vi "Tosca-Setup Connections.vi"(0 "Connect":T2, 2 "Parent VI":refnum<vi>, 7 "config path":path) -> (4 "Connect out":T2, 8 "Canceled?":bool)   [LabVIEW 2020]
uses:
  Classes/Parameters/Connect.ctl
  epl-vi-lib/Utility VIs/Buttons/KCheckmarkBoolean 2.ctl
  Typedefs/Tosca-Locomotion Settings.ctl
  epl-vi-lib/PXI DAQ VIs/TDT VIs/TDT ET VIs/TDT ET-Command Enum.ctl
  epl-vi-lib/TCP VIs/TCP Params.ctl
  epl-vi-lib/TCP VIs/TCP Write.vi
  epl-vi-lib/TCP VIs/TCP-Check Result.vi
  Classes/Parameters/Parameters.lvclass
panel:
  in  "Codes":string
  in  "TCP markers":bool
  in  "LocoTCP":string
  in  "Retrieve data":T1
  in  "Loco Test":cluster{"Ping":bool, "Result":bool}
  in  "Pupil Test":cluster{"Ping":bool, "Result":bool}
  in  "Loco":T1 caption="Record locomotion data"
  in  "Pupil?":T1 caption="Record video"
  out "Ping result":bool
  in  "Ping":bool
  in  "SMP?":T1 caption="Record significant motion pixels (SMP)"
  in  "ET?":T1 caption="Interface with Synapse"
  in  "Cancel":bool
  in  "Apply":bool
  # "Webcam"
  # "Vision display"
  # "Video"
  # "Locomotion"
  # "Neural data"
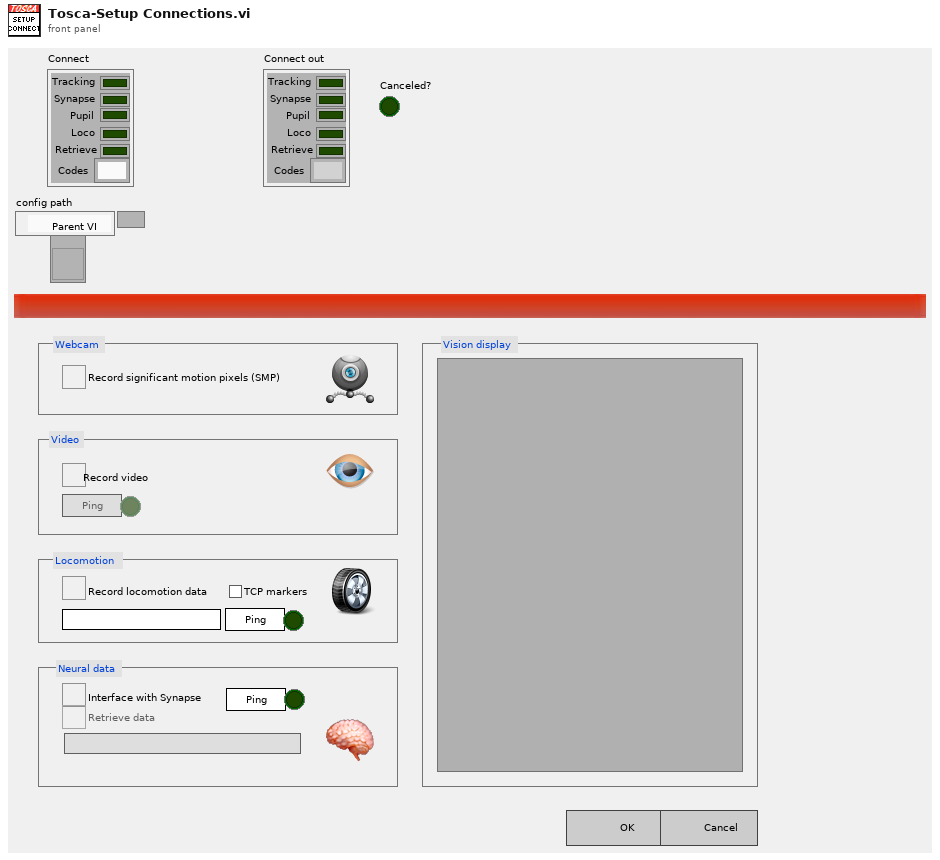
[diagram p1: front panel]
types:
  T1 = typedef "KCheckmarkBoolean 2.ctl" = bool
  T2 = typedef "Parameters.lvclass/Connect.ctl" = cluster{"Tracking":bool, "Synapse":bool, "Pupil":bool, "Loco":bool, "Retrieve":bool, "Codes":string}
  T3 = typedef "TDT ET-Command Enum.ctl" = enum16{"Ping", "Start", "Stop", "NewBlock"}
  T4 = typedef "Tosca-Locomotion Settings.ctl" = cluster{"IP Address":string, "Port":i32, "Send markers":bool}
  T5 = enum8{"Enabled", "Disabled", "Disabled and Grayed Out"}
  T6 = typedef "TCP Params.ctl" = cluster{"IP Address":string, "Port":i32}
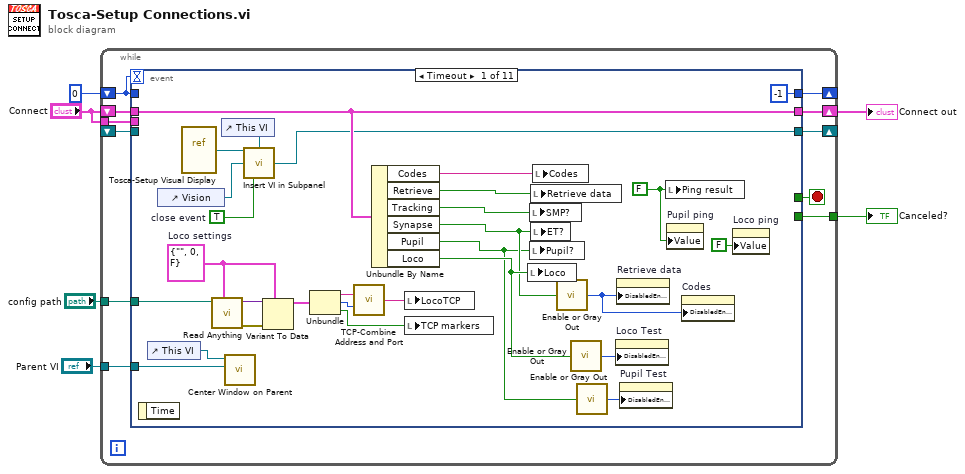
[diagram p0: block diagram]
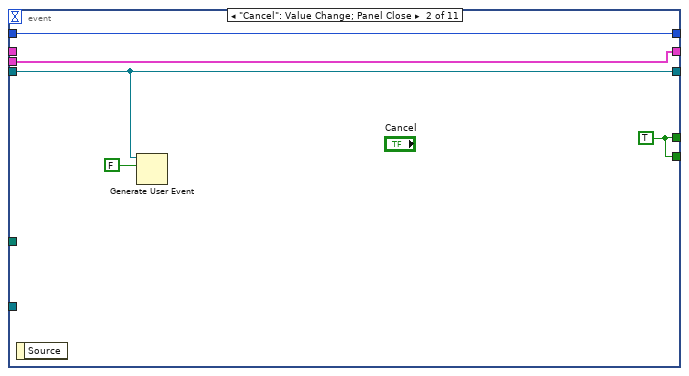
[diagram p2: hidden frame]
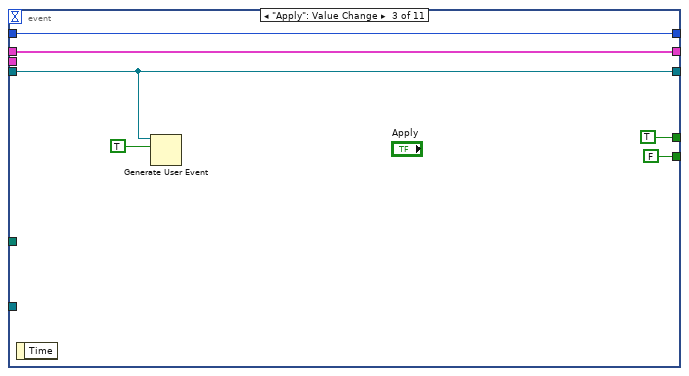
[diagram p3: hidden frame]
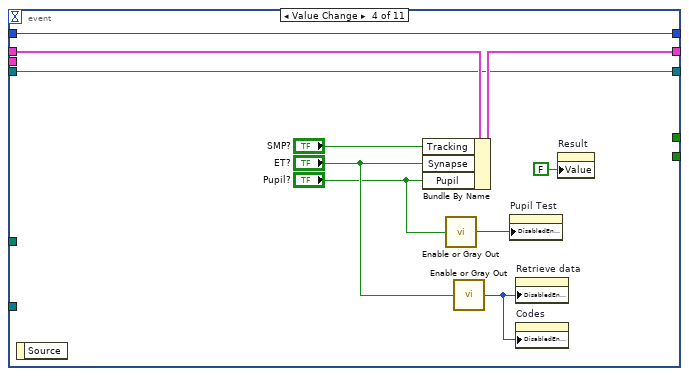
[diagram p4: hidden frame]
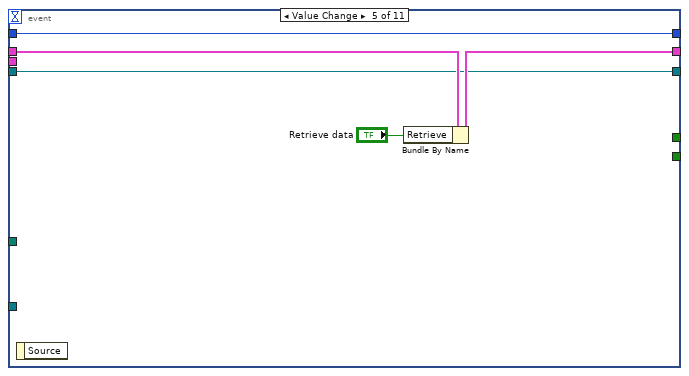
[diagram p5: hidden frame]
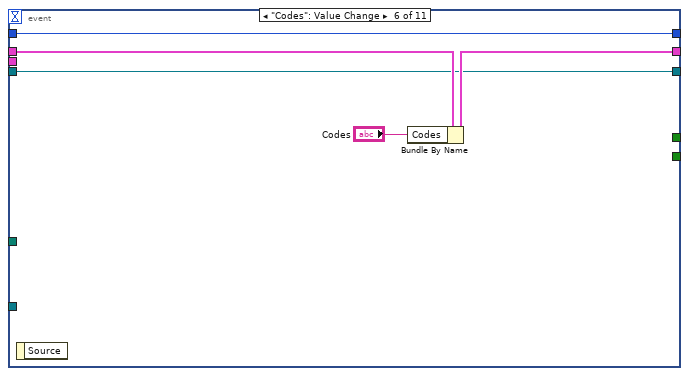
[diagram p6: hidden frame]
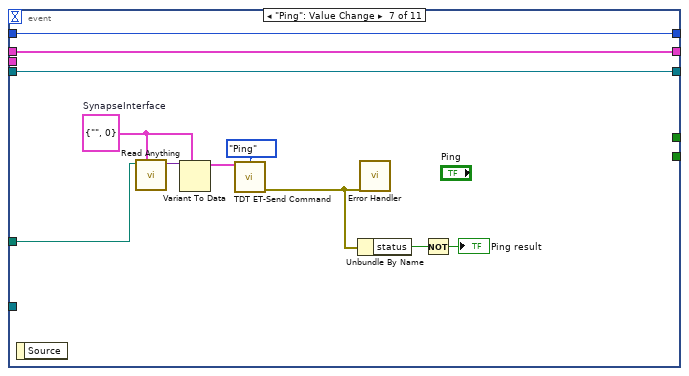
[diagram p7: hidden frame]
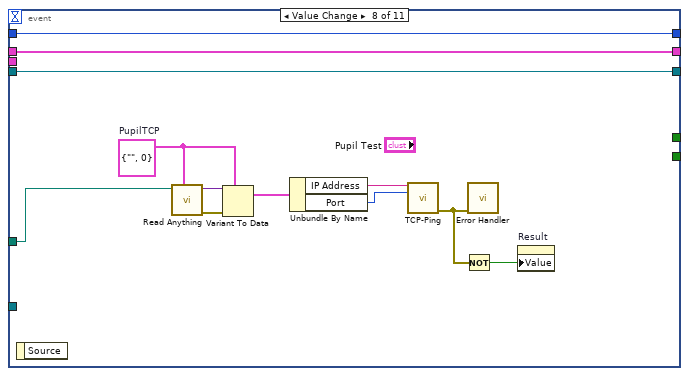
[diagram p8: hidden frame]
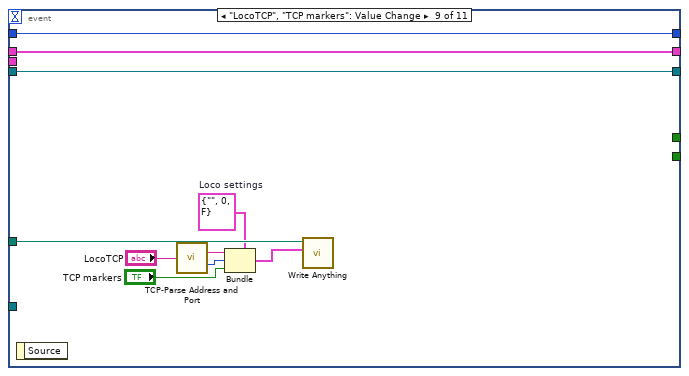
[diagram p9: hidden frame]
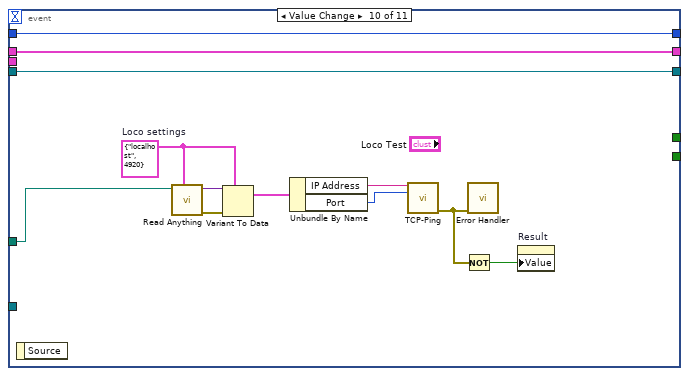
[diagram p10: hidden frame]
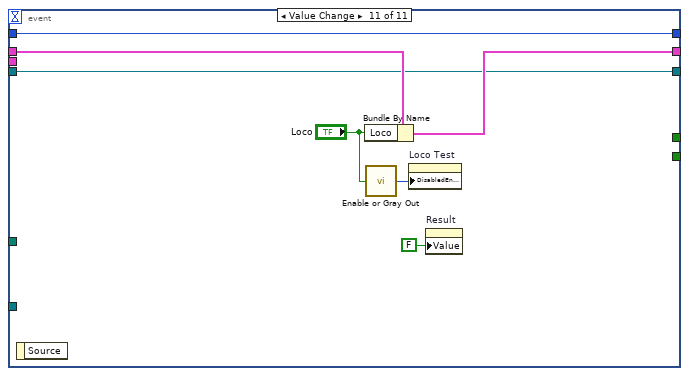
[diagram p11: hidden frame]
diagram:
  n1 = while {
    shift-right: [w17] -> _
    shift-left: 0 -> [w10]
    tunnel: [w13] -> w4
    shift-right: [w15] -> w5
    shift-left: "Connect" -> [w16]
    tunnel: "config path" -> [w12]
    tunnel: "Connect" -> [w11]
    tunnel: "Parent VI" -> [w9]
    shift-right: [w8] -> _
    shift-left: _ -> [w7]
    stop <- w14 stop-if-true
    n2 = event shown="[0] Timeout" {
      selector: _ -> [_ _ _ _ _ _ _ _ _ _ _]
      dyn-events: _ -> [_ _ _ _ _ _ _ _ _ _ _]
      timeout: w10 -> [_ _ _ _ _ _ _ _ _ _ _]
      tunnel: [-1 w49 w54 w64 w72 w77 w83 w100 w110 w122 w129] -> w17
      tunnel: w16 -> [w45 _ w57 w67 w71 w76 w88 w99 w109 w121 w128]
      tunnel: [w45 w50 w57 w66 w70 w75 w88 w99 w109 w121 w127] -> w15
      tunnel: [_ w51 TRUE _ _ _ _ _ _ _ _] -> w14
      tunnel: [_ w51 FALSE _ _ _ _ _ _ _ _] -> w13
      tunnel: w12 -> [w22 _ _ _ _ _ w79 w90 w104 w112 _]
      tunnel: w11 -> [_ w50 _ _ _ _ _ _ _ _ _]
      tunnel: w10 -> [_ w49 w54 w64 w72 w77 w83 w100 w110 w122 w129]
      tunnel: w9 -> [w35 _ _ _ _ _ _ _ _ _ _]
      tunnel: [w29 w48 w53 w59 w68 w74 w82 w89 w108 w111 w123] -> w8
      tunnel: w7 -> [_ w48 w53 w59 w68 w74 w82 w89 w108 w111 w123]
      event Timeout {
        w21 = T4 {"IP Address"="", "Port"=0, "Send markers"=FALSE}  # Loco settings
        w30 = TRUE  # close event
        w40 = FALSE ("Ping result")
        n3 = event-data() -> ()  [unwired: 1 in, 1 out]
        n4 = control-ref of="This VI"() -> (w34:refnum<vi>)
        n5 = control-ref of="Vision"() -> (w32:refnum<vi>)
        n6 = vi-ref "Tosca-Setup Visual Display.vi"() -> (w33:refnum<vi>)
        n7 = call "Read Anything.vi"("Type of Anything"=w21, "Path (dialog)"=w22) -> ("Error Out"=w28:errorcluster, "Anything"=w27:variant)  [unwired: 7 in, 1 out]
        n8 = control-ref of="This VI"() -> (w31:refnum<vi>)
        n9 = call "Center Window on Parent.vi"("Parent VI"=w35, "VI in"=w34) -> ()  [unwired: 8 in, 2 out]
        n10 = call "Insert VI in Subpanel.vi"("VI Ref"=w33, "Parent"=w31, "SubPanel"=w32, "close event"=w30) -> ("close event"=w29:refnum<user-event>)  [unwired: 10 in, 1 out]
        n11 = Variant To Data(error in=w28, type=w21, Variant=w27) -> (data=w26:T4)  [unwired: 1 out]
        n12 = Unbundle(w26) -> ("IP Address"=w25:string, "Port"=w23:i32, "Send markers"=w20:bool)
        n13 = call "TCP-Combine Address and Port.vi"("Address"=w25, "Port"=w23) -> ("Address out"=w24:string)  [unwired: 13 in]
        n14 = Unbundle By Name(w45) -> ("Codes"=w18:string, "Retrieve"=w37:bool, "Tracking"=w44:bool, "Synapse"=w38:bool, "Pupil"=w36:bool, "Loco"=w42:bool)
        n15 = local write "LocoTCP"(w24) -> ()
        n16 = local write "TCP markers"(w20) -> ()
        n17 = local write "Loco"(w42) -> ()
        n18 = local write "SMP?"(w44) -> ()
        n19 = local write "Pupil?"(w36) -> ()
        n20 = local write "Retrieve data"(w37) -> ()
        n21 = local write "ET?"(w38) -> ()
        n22 = local write "Codes"(w18) -> ()
        n23 = call "Enable or Gray Out.vi"("Boolean"=w38) -> ("Disabled"=w19:T5)
        n24 = call "Enable or Gray Out.vi"("Boolean"=w42) -> ("Disabled"=w43:T5)
        n25 = call "Enable or Gray Out.vi"("Boolean"=w36) -> ("Disabled"=w41:T5)
        n26 = property on="Loco Test" class="Clust"("DisabledEnum"=w43) -> ()  [unwired: 2 in, 2 out]
        n27 = property on="Retrieve data" class="Bool (strict)"("DisabledEnum"=w19) -> ()  [unwired: 2 in, 2 out]
        n28 = property on="Pupil Test" class="Clust"("DisabledEnum"=w41) -> ()  [unwired: 2 in, 2 out]
        n29 = local write "Ping result"(w40) -> ()
        n30 = property on="Pupil ping" class="Bool (strict)"("Value"=w40) -> ()  [unwired: 2 in, 2 out]
        n31 = property on="Codes" class="Str"("DisabledEnum"=w19) -> ()  [unwired: 2 in, 2 out]
        n32 = property on="Loco ping" class="Bool (strict)"("Value"=FALSE) -> ()  [unwired: 2 in, 2 out]
      }
      event "Cancel": Value Change; Panel Close {
        w51 = TRUE
        n33 = event-data() -> ()  [unwired: 1 in, 1 out]
        n34 = Generate User Event(user event=w48, event data cluster=FALSE ("event data")) -> ()  [unwired: 2 in, 2 out]
      }
      event "Apply": Value Change {
        n35 = event-data() -> ()  [unwired: 1 in, 1 out]
        n36 = Generate User Event(user event=w53, event data cluster=TRUE ("event data")) -> ()  [unwired: 2 in, 2 out]
      }
      event Value Change {
        n37 = event-data() -> ()  [unwired: 1 in, 1 out]
        n38 = Bundle By Name(cluster=w67, "Tracking"="SMP?", "Synapse"="ET?", "Pupil"="Pupil?") -> (w66:T2)
        n39 = call "Enable or Gray Out.vi"("Boolean"="Pupil?") -> ("Disabled"=w63:T5)
        n40 = call "Enable or Gray Out.vi"("Boolean"="ET?") -> ("Disabled"=w58:T5)
        n41 = property on="Pupil Test" class="Clust"("DisabledEnum"=w63) -> ()  [unwired: 2 in, 2 out]
        n42 = property on="Retrieve data" class="Bool (strict)"("DisabledEnum"=w58) -> ()  [unwired: 2 in, 2 out]
        n43 = property on="Codes" class="Str"("DisabledEnum"=w58) -> ()  [unwired: 2 in, 2 out]
        n44 = property on="Result" class="Bool (strict)"("Value"=FALSE) -> ()  [unwired: 2 in, 2 out]
      }
      event Value Change {
        n45 = event-data() -> ()  [unwired: 1 in, 1 out]
        n46 = Bundle By Name(cluster=w71, "Retrieve"="Retrieve data") -> (w70:T2)
      }
      event "Codes": Value Change {
        n47 = event-data() -> ()  [unwired: 1 in, 1 out]
        n48 = Bundle By Name(cluster=w76, "Codes"="Codes") -> (w75:T2)
      }
      event "Ping": Value Change {
        w80 = T6 {"IP Address"="", "Port"=0}  # SynapseInterface
        n49 = event-data() -> ()  [unwired: 1 in, 1 out]
        n50 = call "Read Anything.vi"("Type of Anything"=w80, "Path (dialog)"=w79) -> ("Anything"=w81:variant)  [unwired: 7 in, 2 out]
        n51 = Variant To Data(type=w80, Variant=w81) -> (data=w78:T6)  [unwired: 1 in, 1 out]
        n52 = call "TDT ET-Send Command.vi"("TCP"=w78, "Command"=TDT_ET-Command_Enum."Ping") -> ("error out"=w84:errorcluster)  [unwired: 11 in, 2 out]
        n53 = Unbundle By Name(w84) -> ("status"=w86:bool)
        n54 = call "Error Handler.vi"("error in (no error)"=w84) -> ()  [unwired: 12 in, 3 out]
        n55 = Not(x=w86) -> (.not. x?=→"Ping result":bool)
      }
      event "Pupil Test.Ping": Value Change {
        w95 = T6 {"IP Address"="", "Port"=0}  # PupilTCP
        n56 = event-data() -> ()  [unwired: 1 in, 1 out]
        n57 = call "Read Anything.vi"("Type of Anything"=w95, "Path (dialog)"=w90) -> ("Error Out"=w97:errorcluster, "Anything"=w96:variant)  [unwired: 7 in, 1 out]
        n58 = Variant To Data(error in=w97, type=w95, Variant=w96) -> (data=w98:T6)  [unwired: 1 out]
        n59 = Unbundle By Name(w98) -> ("IP Address"=w94:string, "Port"=w93:i32)
        n60 = call "TCP-Ping.vi"("IP Address"=w94, "Port"=w93) -> ("error out"=w92:errorcluster)  [unwired: 13 in]
        n61 = Not(x=w92) -> (.not. x?=w91:bool)
        n62 = call "Error Handler.vi"("error in (no error)"=w92) -> ()  [unwired: 12 in, 3 out]
        n63 = property on="Result" class="Bool (strict)"("Value"=w91) -> ()  [unwired: 2 in, 2 out]
      }
      event "LocoTCP", "TCP markers": Value Change {
        w101 = T4 {"IP Address"="", "Port"=0, "Send markers"=FALSE}  # Loco settings
        n64 = event-data() -> ()  [unwired: 1 in, 1 out]
        n65 = call "TCP-Parse Address and Port.vi"("Address in"="LocoTCP") -> ("Address"=w106:string, "Port"=w105:i32)  [unwired: 12 in, 1 out]
        n66 = Bundle(cluster=w101, "IP Address"=w106, "Port"=w105, "Send markers"="TCP markers") -> (w103:T4)
        n67 = call "Write Anything.vi"("Anything"=w103, "Path (dialog)"=w104) -> ()  [unwired: 8 in, 2 out]
      }
      event "Loco Test.Ping": Value Change {
        w117 = T6 {"IP Address"="localhost", "Port"=4920}  # Loco settings
        n68 = event-data() -> ()  [unwired: 1 in, 1 out]
        n69 = call "Read Anything.vi"("Type of Anything"=w117, "Path (dialog)"=w112) -> ("Error Out"=w119:errorcluster, "Anything"=w118:variant)  [unwired: 7 in, 1 out]
        n70 = Variant To Data(error in=w119, type=w117, Variant=w118) -> (data=w120:T6)  [unwired: 1 out]
        n71 = Unbundle By Name(w120) -> ("IP Address"=w116:string, "Port"=w115:i32)
        n72 = call "TCP-Ping.vi"("IP Address"=w116, "Port"=w115) -> ("error out"=w114:errorcluster)  [unwired: 13 in]
        n73 = Not(x=w114) -> (.not. x?=w113:bool)
        n74 = call "Error Handler.vi"("error in (no error)"=w114) -> ()  [unwired: 12 in, 3 out]
        n75 = property on="Result" class="Bool (strict)"("Value"=w113) -> ()  [unwired: 2 in, 2 out]
      }
      event Value Change {
        n76 = event-data() -> ()  [unwired: 1 in, 1 out]
        n77 = Bundle By Name(cluster=w128, "Loco"="Loco") -> (w127:T2)
        n78 = call "Enable or Gray Out.vi"("Boolean"="Loco") -> ("Disabled"=w126:T5)
        n79 = property on="Loco Test" class="Clust"("DisabledEnum"=w126) -> ()  [unwired: 2 in, 2 out]
        n80 = property on="Result" class="Bool (strict)"("Value"=FALSE) -> ()  [unwired: 2 in, 2 out]
      }
    }
  }
  "Connect out" <- w5
  "Canceled?" <- w4
